vi "OE1022D_Auto_Phase.vi"(0 "VISA resource name":refnum<visa-resource-name>, 1 "OE1022D A/B":u8(ring) items=["Channel A", "Channel B"], 5 "错误输入（无错误）":errorcluster) -> (14 "VISA resource name out":refnum<visa-resource-name>, 19 "错误输出":errorcluster)   [LabVIEW 2014]
doc: "Configures the reference source and the internal oscillator."
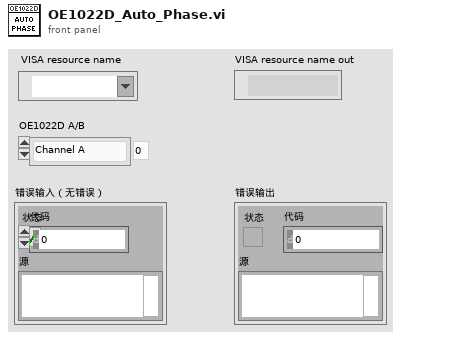
[diagram p1: front panel]
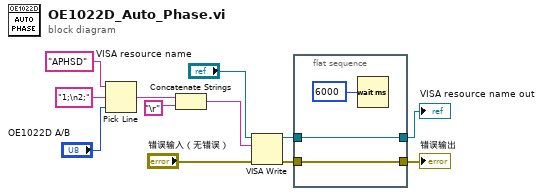
[diagram p0: block diagram]
diagram:
  n1 = Pick Line(string ("")="APHSD", multi-line string="1;\n2;", line index="OE1022D A/B") -> (output string=w7:string)
  n2 = Concatenate Strings(w7, "\r") -> (w9:string)
  n3 = VISA Write(VISA resource name="VISA resource name", write buffer=w9, error in (no error)="错误输入（无错误）") -> (VISA resource name out=w6:refnum<visa-resource-name>, error out=w4:errorcluster)  [unwired: 1 out]
  n4 = flat-sequence {
    tunnel: [w14] -> w5
    tunnel: w6 -> [w14]
    tunnel: w4 -> [w13]
    tunnel: [w13] -> w3
    frame #0 {
      n5 = Wait (ms)(milliseconds to wait=u32 6000 ("等待时间（毫秒）")) -> ()  [unwired: 1 out]
    }
  }
  "VISA resource name out" <- w5
  "错误输出" <- w3
